vi "8-bit video export-Path validator.vi"(8 "error in (no error)":errorcluster, 11 "AVI File Path":path) -> (0 "error out":errorcluster, 3 "Invalid folder":bool)   [LabVIEW 2013]
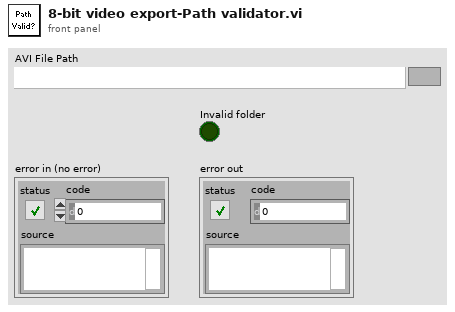
[diagram p1: front panel]
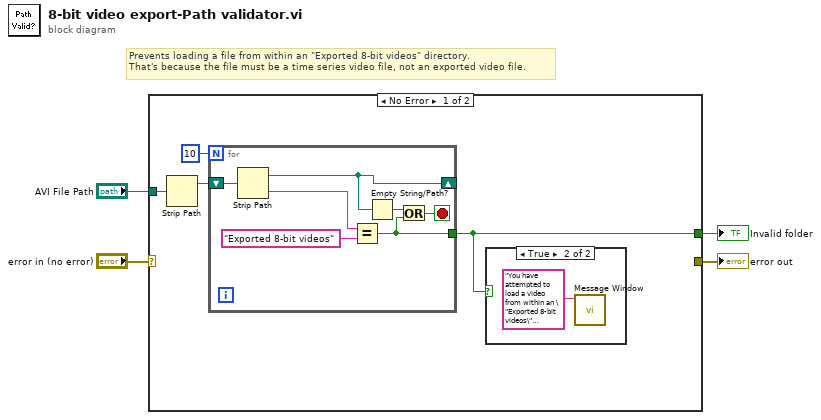
[diagram p0: block diagram]
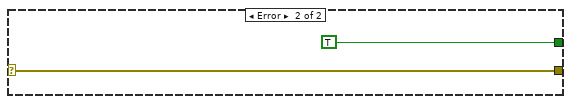
[diagram p3: hidden frame]
diagram:
  # "Prevents loading a file from within an \"Exported 8-bit videos\" directory.\nThat's because the file must be a time series video file, not an exported video file."
  n1 = case shown="No Error" "error in (no error)" {
    selector: "error in (no error)" -> [_ w17]
    tunnel: [_ w17] -> w4
    tunnel: [w5 TRUE] -> w3
    tunnel: "AVI File Path" -> [w6 _]
    frame No Error {
      n2 = Strip Path(path=w6) -> (stripped path=w7:path)  [unwired: 1 out]
      n3 = for {
        N: 10 -> [_]
        shift-right: [w13] -> _
        shift-left: w7 -> [w16]
        tunnel: [w11] -> w5
        stop <- w10 stop-if-true
        n4 = Strip Path(path=w16) -> (stripped path=w13:path, name=w14:string)
        n5 = Equal?(x=w14, y="Exported 8-bit videos") -> (x = y?=w11:bool)
        n6 = Empty String/Path?(string/path=w13) -> (empty?=w12:bool)
        n7 = Or(x=w12, y=w11) -> (x .or. y?=w10:bool)
      }
      n8 = case shown="True" w5 {
        frame False {
        }
        frame True {
          n9 = call "Message Window.vi"("Message string"="You have attempted to load a video from within an \"Exported 8-bit videos\" directory.\n\nYou need to load a time series video instead.") -> ()  [unwired: 10 in, 1 out]
        }
      }
    }
    frame Error {
    }
  }
  "Invalid folder" <- w3
  "error out" <- w4
